vi "Connection Handler.vi"(8 "error in (no error)":errorcluster, 9 "ConnectionID":i32, 10 "References in":T1, 11 "WebSocket Connection in":refnum<class "WebSocket Server.lvclass">) -> (0 "error out":errorcluster)   [LabVIEW 2019]
uses:
  <vilib>/MediaMongrels Ltd/WebSockets/WebSockets/WebSocket Server/WebSocket Server.lvclass
  SubVIs/References.ctl
  <vilib>/MediaMongrels Ltd/Message Queue Helper/ctl_QMH_Message_Typedef.ctl
  Vote Handler/Vote Result.ctl
  Vote Handler/Vote Status Update.ctl
  Vote Handler/VoteMessage.ctl
  <vilib>/MediaMongrels Ltd/Message Queue Helper/MessageQueueHelper.lvlib
panel:
  out "Write":string
  out "Read":string
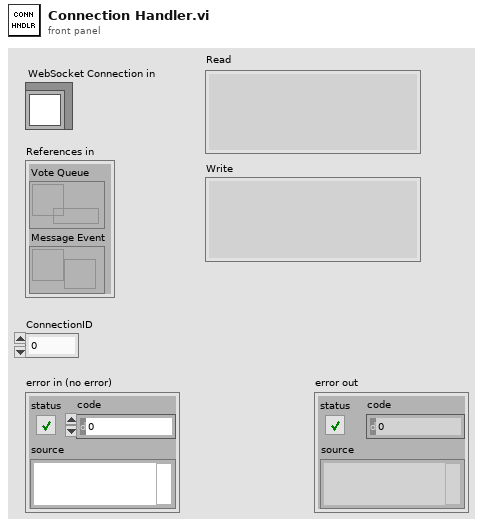
[diagram p1: front panel]
types:
  T1 = typedef "References.ctl" = cluster{"Vote Queue":refnum<queue>, "Message Event":refnum<user-event>}
  T2 = typedef "Vote Result.ctl" = cluster{"Vote":string, "Count":i32}
  T3 = typedef "Vote Status Update.ctl" = cluster{"Vote Frequency (s)":dbl, "Time Remaining":dbl, "# Voters":i32, "Vote Count":i32}
  T4 = typedef "VoteMessage.ctl" = cluster{"VoterID":i32, "VoterInfo":cluster{"VoterName":string, "Ballot":string}}
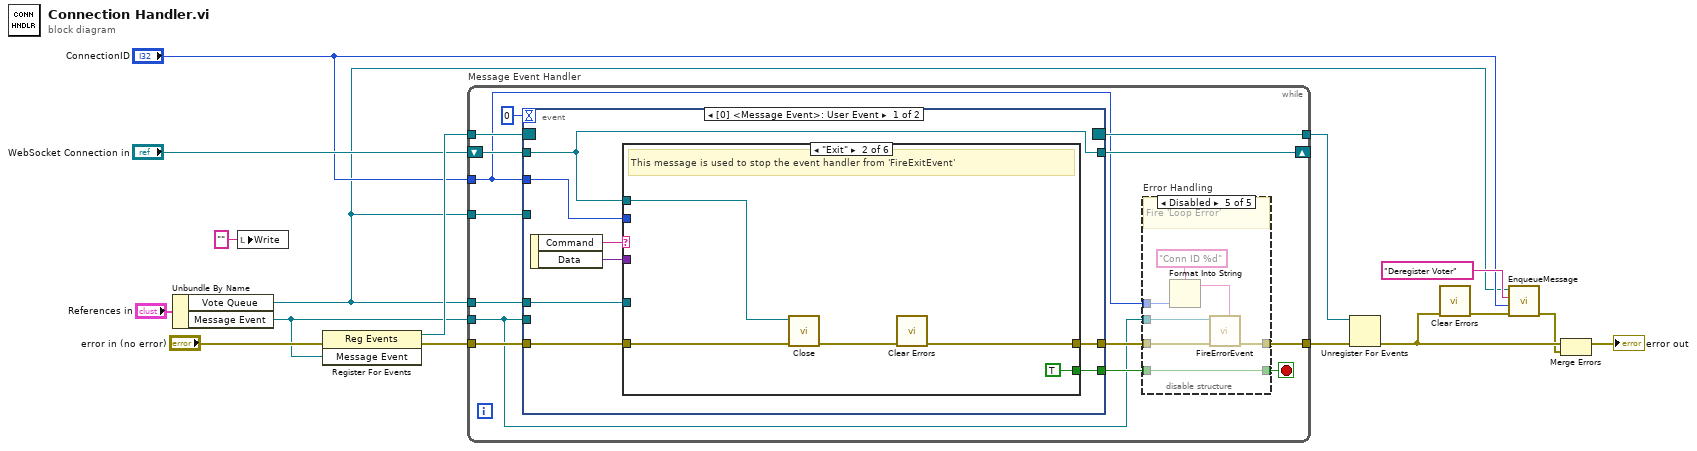
[diagram p0: block diagram]
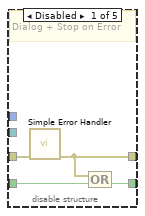
[diagram p2: hidden frame]
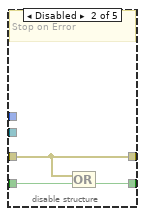
[diagram p3: hidden frame]
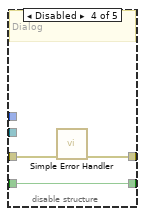
[diagram p5: hidden frame]
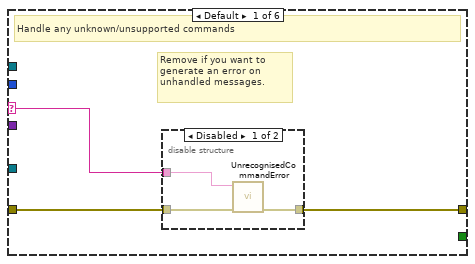
[diagram p6: hidden frame]
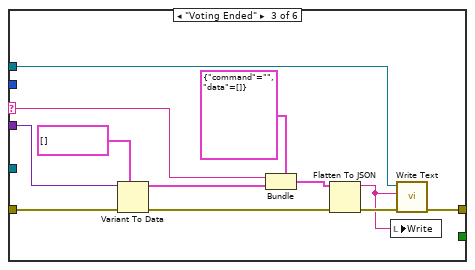
[diagram p8: hidden frame]
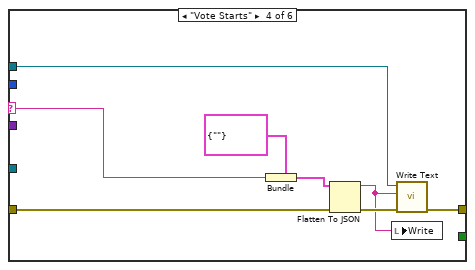
[diagram p9: hidden frame]
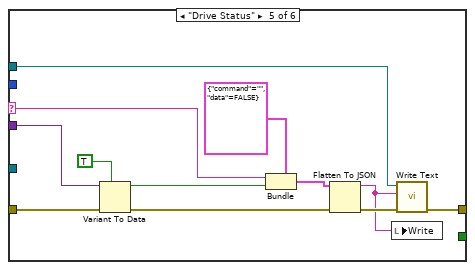
[diagram p10: hidden frame]
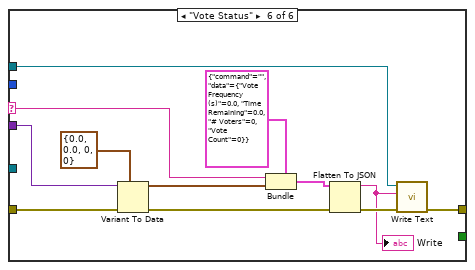
[diagram p11: hidden frame]
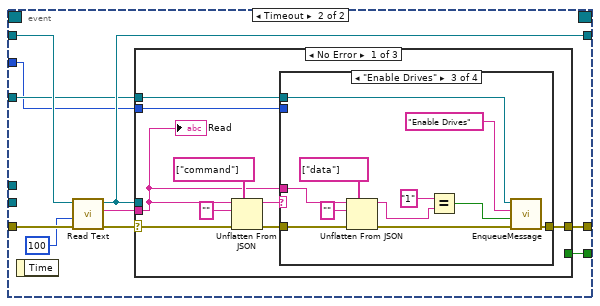
[diagram p12: hidden frame]
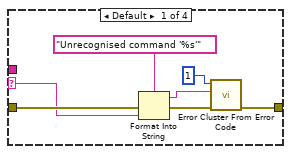
[diagram p13: hidden frame]
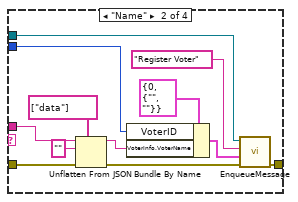
[diagram p14: hidden frame]
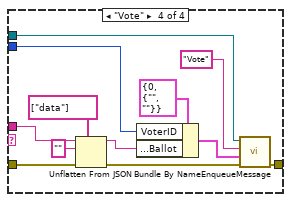
[diagram p15: hidden frame]
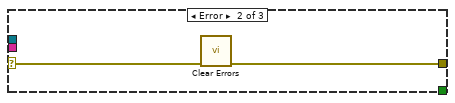
[diagram p16: hidden frame]
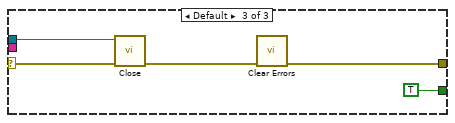
[diagram p17: hidden frame]
diagram:
  n1 = Unbundle By Name("References in") -> ("Vote Queue"=w1:refnum<queue>, "Message Event"=w9:refnum<user-event>)
  n2 = local write "Write"("" ("Write")) -> ()
  n3 = register-events(error in="error in (no error)", w9) -> (reference out=w14:refnum<event-registration>, error out=w13:errorcluster)  [unwired: 1 in]
  n4 = while "Message Event Handler" {
    tunnel: w13 -> [w28]
    tunnel: w14 -> [w30]
    tunnel: [w29] -> w15
    tunnel: [w24] -> w16
    tunnel: w9 -> [w23]
    shift-right: [w20] -> _
    shift-left: "WebSocket Connection in" -> [w21]
    tunnel: "ConnectionID" -> [w18]
    tunnel: w1 -> [w19]
    tunnel: w1 -> [w17]
    stop <- w25 stop-if-true
    n5 = event shown="[0] <Message Event>: User Event" {
      selector: w30 -> [_ _]
      dyn-events: [_ _] -> w29
      timeout: 0 -> [_ _]
      tunnel: [w54 w119] -> w26
      tunnel: w28 -> [w55 w123]
      tunnel: [w53 w117] -> w27
      tunnel: w23 -> [_ _]
      tunnel: w21 -> [w52 w121]
      tunnel: [w52 w116] -> w20
      tunnel: w18 -> [w51 w114]
      tunnel: w19 -> [_ w115]
      tunnel: w17 -> [w50 _]
      event User Event {
        n6 = event-data() -> ("Command"=w57:string, "Data"=w56:variant)  [unwired: 1 in]
        n7 = case shown="\"Exit\"" w57 {
          selector: w57 -> [w58 _ w71 w83 w95 w102]
          tunnel: w56 -> [_ _ w77 _ w92 w109]
          tunnel: w55 -> [w60 w68 w81 w84 w96 w113]
          tunnel: [w59 w65 w80 w89 w101 w112] -> w54
          tunnel: [_ TRUE _ _ _ _] -> w53
          tunnel: w52 -> [_ w66 w79 w88 w100 w111]
          tunnel: w51 -> [_ _ _ _ _ _]
          tunnel: w50 -> [_ _ _ _ _ _]
          frame Default {
            # "Remove if you want to generate an error on unhandled messages."
            # "Handle any unknown/unsupported commands"
            n8 = disable-structure shown="Disabled" {
              disable-tunnel: w60 -> [w62 w64]
              disable-tunnel: [w63 w64] -> w59
              disable-tunnel: w58 -> [w61 _]
              frame Disabled {
                n9 = call <vilib>:"UnrecognisedCommandError.vi"("error in (no error)"=w62, "Command"=w61) -> ("error out"=w63:errorcluster)  [unwired: 9 in]
              }
              frame Enabled {
              }
            }
          }
          frame "Exit" {
            # "This message is used to stop the event handler from 'FireExitEvent'"
            n10 = call-dynamic "Close.vi"("error in (no error)"=w68, "WebSocket in"=w66) -> ("error out"=w67:errorcluster)  [unwired: 9 in]
            n11 = call <vilib>:"Clear Errors.vi"("error in (no error)"=w67) -> ("error out"=w65:errorcluster)  [unwired: 5 in, 1 out]
          }
          frame "Voting Ended" {
            n12 = Variant To Data(error in=w81, type=T2[] [] ("Array"), Variant=w77) -> (data=w75:T2[], error out=w78:errorcluster)
            n13 = Bundle(cluster=cluster{"command":string, "data":T2[]} {"command"="", "data"=[]}, "command"=w71, "data"=w75) -> (w72:cluster{"command":string, "data":T2[]})
            n14 = Flatten To JSON(anything=w72, error in (no error)=w78) -> (JSON string=w70:string, 11:w74:errorcluster)  [unwired: 1 in]
            n15 = local write "Write"(w70) -> ()
            n16 = call-dynamic "Write Text.vi"("error in (no error)"=w74, "String Data"=w70, "WebSocket in"=w79) -> ("error out"=w80:errorcluster)  [unwired: 7 in, 1 out]
          }
          frame "Vote Starts" {
            n17 = Bundle(cluster=cluster{"command":string} {"command"=""}, "command"=w83) -> (w85:cluster{"command":string})
            n18 = Flatten To JSON(anything=w85, error in (no error)=w84) -> (JSON string=w82:string, 11:w87:errorcluster)  [unwired: 1 in]
            n19 = local write "Write"(w82) -> ()
            n20 = call-dynamic "Write Text.vi"("error in (no error)"=w87, "String Data"=w82, "WebSocket in"=w88) -> ("error out"=w89:errorcluster)  [unwired: 7 in, 1 out]
          }
          frame "Drive Status" {
            n21 = Variant To Data(error in=w96, type=TRUE, Variant=w92) -> (data=w90:bool, error out=w93:errorcluster)
            n22 = Bundle(cluster=cluster{"command":string, "data":bool} {"command"="", "data"=FALSE}, "command"=w95, "data"=w90) -> (w97:cluster{"command":string, "data":bool})
            n23 = Flatten To JSON(anything=w97, error in (no error)=w93) -> (JSON string=w94:string, 11:w99:errorcluster)  [unwired: 1 in]
            n24 = local write "Write"(w94) -> ()
            n25 = call-dynamic "Write Text.vi"("error in (no error)"=w99, "String Data"=w94, "WebSocket in"=w100) -> ("error out"=w101:errorcluster)  [unwired: 7 in, 1 out]
          }
          frame "Vote Status" {
            n26 = Variant To Data(error in=w113, type=T3 {"Vote Frequency (s)"=0.0, "Time Remaining"=0.0, "# Voters"=0, "Vote Count"=0} ("cluster"), Variant=w109) -> (data=w108:T3, error out=w110:errorcluster)
            n27 = Bundle(cluster=cluster{"command":string, "data":T3} {"command"="", "data"={"Vote Frequency (s)"=0.0, "Time Remaining"=0.0, "# Voters"=0, "Vote Count"=0}}, "command"=w102, "data"=w108) -> (w105:cluster{"command":string, "data":T3})
            n28 = Flatten To JSON(anything=w105, error in (no error)=w110) -> (JSON string=w104:string, 11:w107:errorcluster)  [unwired: 1 in]
            "Write" <- w104
            n29 = call-dynamic "Write Text.vi"("error in (no error)"=w107, "String Data"=w104, "WebSocket in"=w111) -> ("error out"=w112:errorcluster)  [unwired: 7 in, 1 out]
          }
        }
      }
      event Timeout {
        n30 = event-data() -> ()  [unwired: 1 in, 1 out]
        n31 = call-dynamic "Read Text.vi"("error in (no error)"=w123, "timeout ms (5000)"=100, "WebSocket in"=w121) -> ("error out"=w120:errorcluster, "Data"=w118:string, "WebSocket out"=w116:refnum<class "WebSocket Server.lvclass">)  [unwired: 6 in]
        n32 = case shown="No Error" w120 {
          selector: w120 -> [w132 w176 w180]
          tunnel: [w127 w175 w177] -> w119
          tunnel: w118 -> [w126 _ _]
          tunnel: w116 -> [_ _ w179]
          tunnel: [_ _ TRUE] -> w117
          tunnel: w115 -> [w125 _ _]
          tunnel: w114 -> [w124 _ _]
          frame No Error {
            n33 = Unflatten From JSON(path=string[] ["command"], JSON string=w126, type and defaults="", error in (no error)=w132) -> (value=w128:string, error out=w129:errorcluster)  [unwired: 3 in]
            n34 = case shown="\"Enable Drives\"" w128 {
              selector: w128 -> [w136 _ _ _]
              tunnel: w129 -> [w139 w151 w162 w174]
              tunnel: [w138 w146 w158 w169] -> w127
              tunnel: w126 -> [_ w150 w161 w173]
              tunnel: w125 -> [_ w145 w157 w168]
              tunnel: w124 -> [_ w142 _ w165]
              frame Default {
                n35 = Format Into String(format string="Unrecognised command '%s'", error in=w139, w136) -> (resulting string=w134:string, error out=w137:errorcluster)  [unwired: 1 in]
                n36 = call <vilib>:"Error Cluster From Error Code.vi"("error in (no error)"=w137, "error message (\"\")"=w134, "error code (0)"=1) -> ("error out"=w138:errorcluster)  [unwired: 6 in]
              }
              frame "Name" {
                n37 = Unflatten From JSON(path=string[] ["data"], JSON string=w150, type and defaults="", error in (no error)=w151) -> (value=w141:string, error out=w147:errorcluster)  [unwired: 3 in]
                n38 = Bundle By Name(cluster=T4 {"VoterID"=0, "VoterInfo"={"VoterName"="", "Ballot"=""}}, "VoterID"=w142, "VoterInfo.VoterName"=w141) -> (w140:T4)
                n39 = call <vilib>:"EnqueueMessage.vi"("error in (no error)"=w147, "Data"=w140, "Command"="Register Voter", "Message Queue in"=w145) -> ("error out"=w146:errorcluster)  [unwired: 5 in, 2 out]
              }
              frame "Enable Drives" {
                n40 = Unflatten From JSON(path=string[] ["data"], JSON string=w161, type and defaults="", error in (no error)=w162) -> (value=w154:string, error out=w159:errorcluster)  [unwired: 3 in]
                n41 = Equal?(x="1", y=w154) -> (x = y?=w153:bool)
                n42 = call <vilib>:"EnqueueMessage.vi"("error in (no error)"=w159, "Data"=w153, "Command"="Enable Drives", "Message Queue in"=w157) -> ("error out"=w158:errorcluster)  [unwired: 5 in, 2 out]
              }
              frame "Vote" {
                n43 = Unflatten From JSON(path=string[] ["data"], JSON string=w173, type and defaults="", error in (no error)=w174) -> (value=w164:string, error out=w170:errorcluster)  [unwired: 3 in]
                n44 = Bundle By Name(cluster=T4 {"VoterID"=0, "VoterInfo"={"VoterName"="", "Ballot"=""}}, "VoterID"=w165, "VoterInfo.Ballot"=w164) -> (w163:T4)
                n45 = call <vilib>:"EnqueueMessage.vi"("error in (no error)"=w170, "Data"=w163, "Command"="Vote", "Message Queue in"=w168) -> ("error out"=w169:errorcluster)  [unwired: 5 in, 2 out]
              }
            }
            "Read" <- w126
          }
          frame Error {
            n46 = call <vilib>:"Clear Errors.vi"("error in (no error)"=w176) -> ("error out"=w175:errorcluster)  [unwired: 5 in, 1 out]
          }
          frame Default {
            n47 = call-dynamic "Close.vi"("error in (no error)"=w180, "WebSocket in"=w179) -> ("error out"=w178:errorcluster)  [unwired: 9 in]
            n48 = call <vilib>:"Clear Errors.vi"("error in (no error)"=w178) -> ("error out"=w177:errorcluster)  [unwired: 5 in, 1 out]
          }
        }
      }
    }
    n49 = disable-structure "Error Handling" shown="Disabled" {
      disable-tunnel: w27 -> [w34 w37 w38 w41 w46]
      disable-tunnel: w26 -> [w33 w35 w39 w42 w49]
      disable-tunnel: [w32 w36 w38 w41 w46] -> w25
      disable-tunnel: [w31 w35 w39 w40 w47] -> w24
      disable-tunnel: w23 -> [_ _ _ _ w48]
      disable-tunnel: w18 -> [_ _ _ _ w45]
      frame Disabled {
        # "Dialog + Stop on Error"
        n50 = call <vilib>:"Simple Error Handler.vi"("error in (no error)"=w33) -> ("error out"=w31:errorcluster)  [unwired: 4 in, 4 out]
        n51 = Compound Arithmetic op=OR(w31, w34) -> (w32:bool)
      }
      frame Disabled {
        # "Stop on Error"
        n52 = Compound Arithmetic op=OR(w35, w37) -> (w36:bool)
      }
      frame Enabled {
        # "Continue on Error"
      }
      frame Disabled {
        # "Dialog"
        n53 = call <vilib>:"Simple Error Handler.vi"("error in (no error)"=w42) -> ("error out"=w40:errorcluster)  [unwired: 4 in, 4 out]
      }
      frame Disabled {
        # "Fire 'Loop Error'"
        n54 = Format Into String(format string="Conn ID %d", w45) -> (resulting string=w43:string)  [unwired: 2 in, 1 out]
        n55 = call <vilib>:"FireErrorEvent.vi"("Source"=w43, "error in (no error)"=w49, "Message Event in"=w48) -> ("error out"=w47:errorcluster)  [unwired: 8 in]
      }
    }
  }
  n56 = Unregister For Events(event registration refnum=w15, error in=w16) -> (error out=w4:errorcluster)
  n57 = call <vilib>:"Clear Errors.vi"("error in (no error)"=w4) -> ("error out"=w5:errorcluster)  [unwired: 5 in, 1 out]
  n58 = call <vilib>:"EnqueueMessage.vi"("error in (no error)"=w5, "Data"="ConnectionID", "Command"="Deregister Voter", "Message Queue in"=w1) -> ("error out"=w2:errorcluster)  [unwired: 5 in, 2 out]
  n59 = Merge Errors(w4, w2) -> (→"error out":errorcluster)
